vi "GetComputerNameA.vi"() -> (3 "Computer Name":string)   [LabVIEW 2021]
uses:
  Windows/System32/kernel32.dll
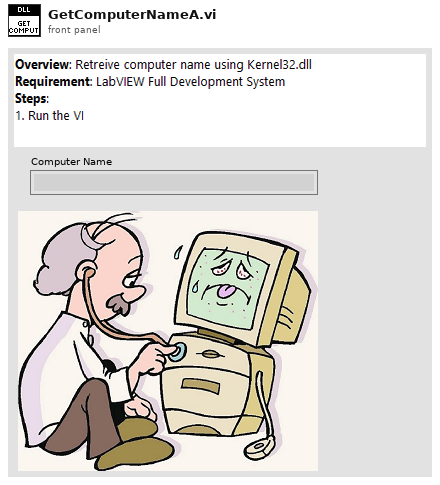
[diagram p1: front panel]
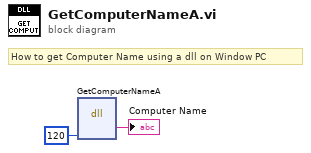
[diagram p0: block diagram]
diagram:
  # "How to get Computer Name using a dll on Window PC"
  n1 = dll-call lib="C:/Windows/System32/kernel32.dll" fn="GetComputerNameA"("lpnSize"=120) -> ("lpbuffer"=→"Computer Name":string)  [unwired: 6 in, 2 out]
